vi "Wave1D_Cal U1.vi"(11 "Wave1D Data In":T1 {"BC"."End X"."type" items=["Dirichlet", "Neumann"]; "BC"."Start X"."type" items=["Dirichlet", "Neumann"]}) -> (3 "Wave1D Data Out":T1 {"BC"."End X"."type" items=["Dirichlet", "Neumann"]; "BC"."Start X"."type" items=["Dirichlet", "Neumann"]})   [LabVIEW 2020, in "NI_PDE.lvlib"]
uses:
  <vilib>/gmath/NI_PDE.lvlib
  <vilib>/gmath/pde.llb/Wave1D/Wave1D_Data.ctl
  <vilib>/gmath/pde.llb/Common/PDE_BC Type.ctl
  <vilib>/Analysis/Matrix/Datatypes/RealMatrix.ctl
  <vilib>/Analysis/Matrix/NI_Matrix.lvlib
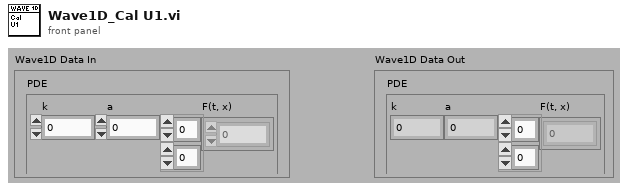
[diagram p1: front panel]
types:
  T1 = typedef "NI_PDE.lvlib/Wave1D_Data.ctl" = cluster{"PDE":cluster{"k":dbl, "a":dbl, "F(t, x)":dbl[][]}, "Domain":cluster{"t":cluster{"initial t":dbl, "final t":dbl, "# of t-points":i32}, "x":cluster{"start x":dbl, "end x":dbl, "# of x-points":i32}, "delta":cluster{"delta t":dbl, "delta x":dbl}}, "BC":cluster{"Start X":cluster{"type":T2, "Value":dbl[]}, "End X":cluster{"type":T2, "Value":dbl[]}}, "IC":cluster{"Value":dbl[], "Derivative":dbl[]}, "A":cluster{"Sub Diag":dbl[], "Diag":dbl[], "Super Diag":dbl[], "A":T3}, "LU of A":cluster{"L":dbl[], "U":cluster{"Diag":dbl[], "Super Diag":dbl[], "2nd Super Diag":dbl[]}, "Pivot":i32[]}, "State":cluster{"U":dbl[], "AU":dbl[], "Old AU":dbl[], "start index":i32, "length":i32}}
  T2 = typedef "NI_PDE.lvlib/PDE_BC Type.ctl" = i32
  T3 = typedef "NI_Matrix.lvlib/RealMatrix.ctl" = dbl[][]
  T4 = cluster{"Sub Diag":dbl[], "Diag":dbl[], "Super Diag":dbl[], "A":T3}
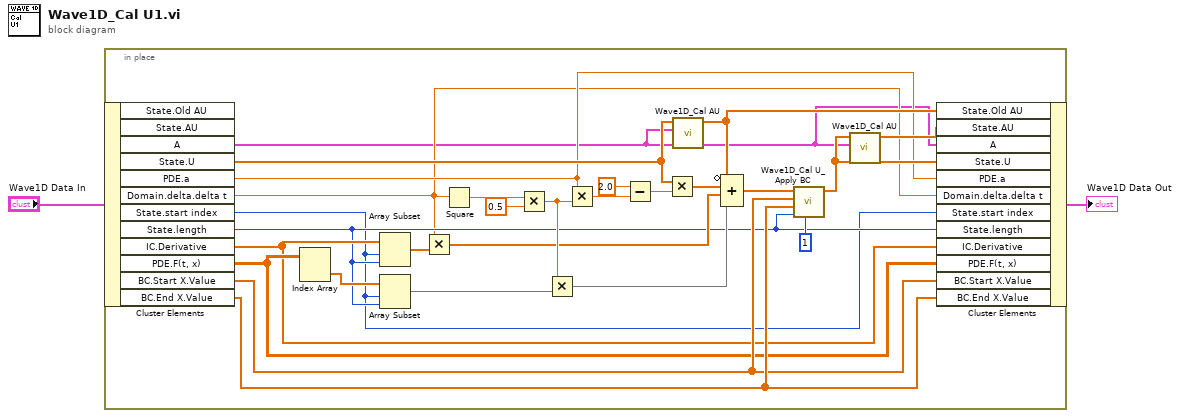
[diagram p0: block diagram]
diagram:
  n1 = in-place {
    n2 = in-place-cluster #1("Wave1D Data In") -> ("A"=w3:T4, "State.U"=w15:dbl[], "PDE.a"=w5:dbl, "Domain.delta.delta t"=w4:dbl, "State.start index"=w6:i32, "State.length"=w7:i32, "IC.Derivative"=w8:dbl[], "PDE.F(t, x)"=w9:dbl[][], "BC.Start X.Value"=w10:dbl[], "BC.End X.Value"=w11:dbl[])  [unwired: 2 out]
    n3 = Index Array(array=w9) -> (element=w23:dbl[])  [unwired: 2 in]
    n4 = Array Subset(array=w8, index=w6, length=w7) -> (w24:dbl[])
    n5 = Array Subset(array=w23, index=w6, length=w7) -> (w22:dbl[])
    n6 = Multiply(x=w4, y=w24) -> (x*y=w19:dbl[])
    n7 = Square(x=w4) -> (x^2=w26:dbl)
    n8 = Multiply(x=w26, y=0.5 ("value")) -> (x*y=w21:dbl)
    n9 = Multiply(x=w21, y=w22) -> (x*y=w18:dbl[])
    n10 = Multiply(x=w5, y=w21) -> (x*y=w29:dbl)
    n11 = Subtract(x=2.0, y=w29) -> (x-y=w27:dbl)
    n12 = Multiply(x=w15, y=w27) -> (x*y=w20:dbl[])
    n13 = call <vilib>:"Wave1D_Cal AU.vi"("A"=w3, "U"=w15) -> ("AU"=w12:dbl[])  [unwired: 9 out]
    n14 = Compound Arithmetic op=ADD(invert w12, w20, w19, w18) -> (w17:dbl[])
    n15 = call <vilib>:"Wave1D_Cal U_Apply BC.vi"("time step"=1, "length"=w7, "End X Value"=w11, "Start X Value"=w10, "U In"=w17) -> ("U Out"=w14:dbl[])  [unwired: 6 out]
    n16 = call <vilib>:"Wave1D_Cal AU.vi"("A"=w3, "U"=w14) -> ("AU"=w13:dbl[])  [unwired: 9 out]
    n17 = in-place-cluster #1("State.Old AU"=w12, "State.AU"=w13, "A"=w3, "State.U"=w14, "PDE.a"=w5, "Domain.delta.delta t"=w4, "State.start index"=w6, "State.length"=w7, "IC.Derivative"=w8, "PDE.F(t, x)"=w9, "BC.Start X.Value"=w10, "BC.End X.Value"=w11) -> (→"Wave1D Data Out":T1)
  }
